vi "SVPO Peak Level (N Ch DBL Array).vi"(6 "restart averaging? (F)":bool, 10 "sampling rate [Hz]":dbl=1.0, 11 "scaled signals [EU]":dbl[][](array[numeric])) -> (1 "minimum levels [EU]":dbl[](array[numeric]), 2 "maximum levels [EU]":dbl[](array[numeric]), 3 "peak levels [EU]":dbl[](array[numeric]), 4 "durations [s]":dbl[](array[numeric]))   [LabVIEW 2017, in "SoundVib_VibrationLevel.lvlib"]
doc: "Uses a peak detector and computes the level of scaled time waveform signals and scaled array signals. <B>scaled signal [EU]</B> should have a zero DC component. You can attenuate the DC component with hardware AC-coupling filters and with software high-pass filters. Use this VI on embedded targets that have limited computational resources. Wire data to the scaled signal [EU] input to determine the polymorphic instance to use or manually select the instance."
uses:
  <vilib>/addons/Sound and Vibration/svt_Level/SoundVib_VibrationLevel.lvlib
  <vilib>/addons/_NISVFA/_Shared subVIs/Controls/svc_Peak Level State.ctl
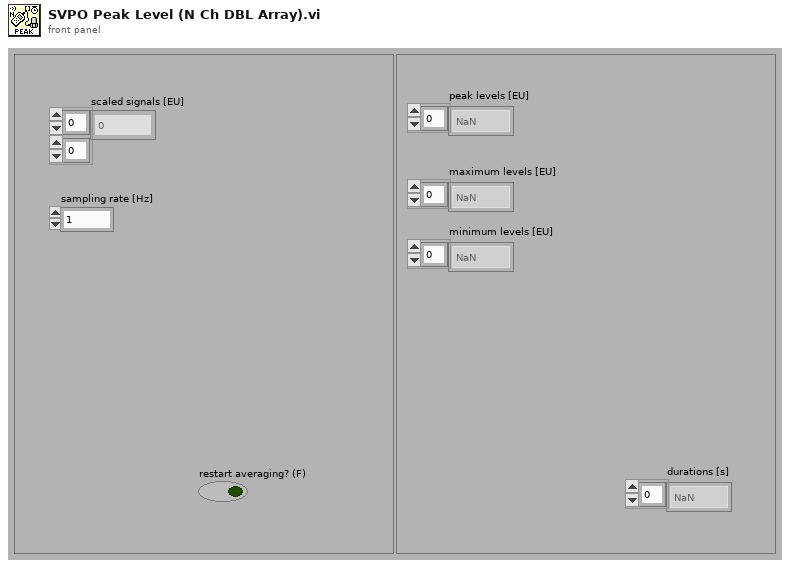
[diagram p1: front panel]
types:
  T1 = typedef "svc_Peak Level State.ctl" = cluster{"historical max":dbl, "historical min":dbl, "cumulative size":u64, "timestamp":timestamp}
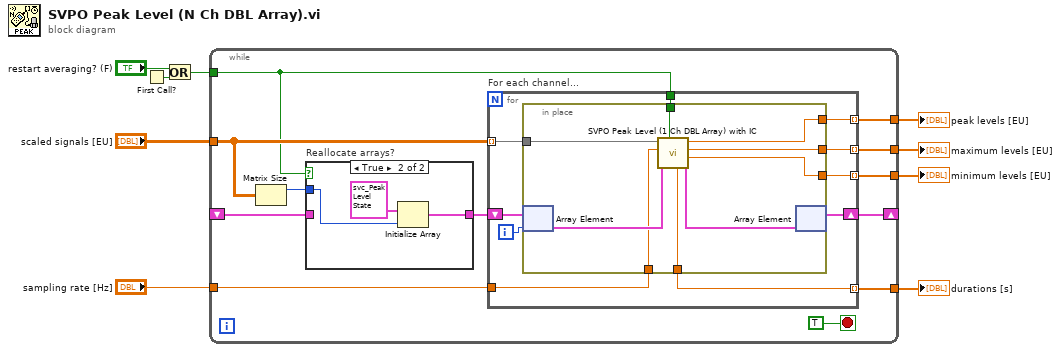
[diagram p0: block diagram]
diagram:
  n1 = First Call?() -> (First Call?: T/F=w8:bool)
  n2 = Or(x="restart averaging? (F)", y=w8) -> (x .or. y?=w5:bool)
  n3 = while {
    tunnel: w5 -> [w10]
    tunnel: "scaled signals [EU]" -> [w12]
    tunnel: [w21] -> w9
    shift-right: [w19] -> _
    shift-left: _ -> [w13]
    tunnel: [w17] -> w4
    tunnel: "sampling rate [Hz]" -> [w16]
    tunnel: [w15] -> w2
    tunnel: [w14] -> w1
    stop <- TRUE stop-if-true
    n4 = Matrix Size(0:w12) -> (1:w11:i32)  [unwired: 1 out]
    n5 = case "Reallocate arrays?" shown="True" w10 {
      tunnel: [w22 w25] -> w18
      tunnel: w13 -> [w22 _]
      tunnel: w11 -> [_ w23]
      frame False {
      }
      frame True {
        n6 = Initialize Array(T1 {"historical max"=-inf, "historical min"=inf, "cumulative size"=0, "timestamp"=timestamp(0 s since 1904-01-01)} ("Initial Conditions"), w23) -> (w25:T1[])
      }
    }
    n7 = for "For each channel..." {
      tunnel: [w29] -> w21 mode=indexing
      tunnel: w10 -> [w35]
      tunnel: w12 -> [w34] mode=indexing
      tunnel: w16 -> [w28]
      shift-right: [w32] -> w19
      shift-left: w18 -> [w33]
      tunnel: [w30] -> w17 mode=indexing
      tunnel: [w27] -> w15 mode=indexing
      tunnel: [w26] -> w14 mode=indexing
      i -> [w31]
      n8 = in-place {
        in-place-border: w35 -> [w37]
        in-place-border: w34 -> [w41]
        in-place-border: [w42] -> w30
        in-place-border: [w40] -> w29
        in-place-border: w28 -> [w39]
        in-place-border: [w38] -> w27
        in-place-border: [w36] -> w26
        n9 = in-place-array #1(w33, w31) -> (w44:T1)
        n10 = call <vilib>:"SVPO Peak Level (1 Ch DBL Array) with IC.vi"("restart averaging? (F)"=w37, "initial conditions"=w44, "sampling rate [Hz]"=w39, "scaled signal [EU]"=w41) -> ("final conditions"=w43:T1, "minimum level [EU]"=w36:dbl, "maximum level [EU]"=w38:dbl, "peak level [EU]"=w42:dbl, "duration [s]"=w40:dbl)  [unwired: 3 in]
        n11 = in-place-array #1(w43) -> (w32:T1[])  [unwired: 1 out]
      }
    }
  }
  "peak levels [EU]" <- w4
  "maximum levels [EU]" <- w2
  "minimum levels [EU]" <- w1
  "durations [s]" <- w9
